vi "Move map.vi"(6 "MAP3":refnum<vi>, 7 "revise":u32=20, 8 "error in":errorcluster, 9 "MAP2":refnum<vi>, 10 "MAP1":refnum<vi>, 11 "Boolean in":refnum<vi>) -> (0 "error out":errorcluster)   [LabVIEW 2010]
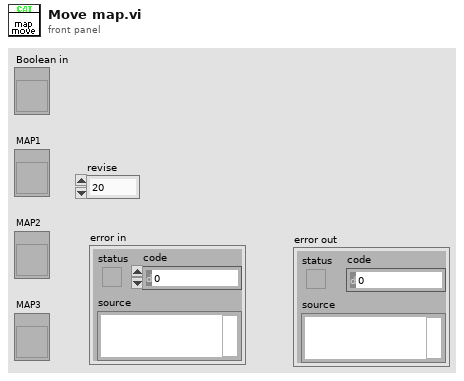
[diagram p1: front panel]
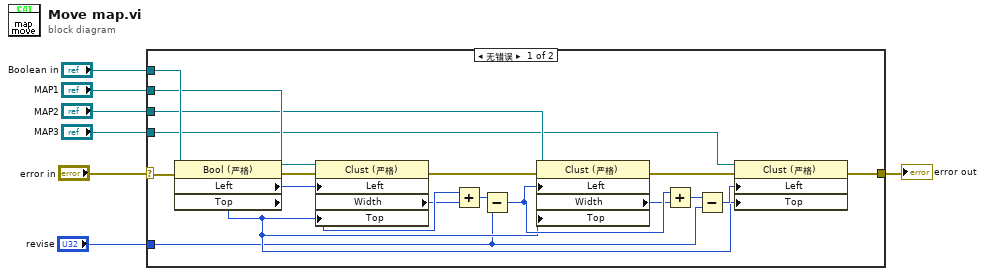
[diagram p0: block diagram]
diagram:
  n1 = case shown="无错误" "error in" {
    selector: "error in" -> [w9 w26]
    tunnel: [w21 w26] -> w7
    tunnel: "Boolean in" -> [w20 _]
    tunnel: "MAP1" -> [w12 _]
    tunnel: "MAP2" -> [w11 _]
    tunnel: "MAP3" -> [w10 _]
    tunnel: "revise" -> [w8 _]
    frame No Error {
      n2 = property class="Bool (严格)"(reference=w20, error in=w9) -> (error out=w15:errorcluster, "Left"=w19:i32, "Top"=w16:i32)  [unwired: 1 out]
      n3 = property class="Clust (严格)"(reference=w12, error in=w15, "Left"=w19, "Top"=w16) -> (error out=w14:errorcluster, "Width"=w18:u32)  [unwired: 1 out]
      n4 = Add(x=w19, y=w18) -> (x+y=w22:u32)
      n5 = Subtract(x=w22, y=w8) -> (x-y=w23:u32)
      n6 = property class="Clust (严格)"(reference=w11, error in=w14, "Left"=w23, "Top"=w16) -> (error out=w13:errorcluster, "Width"=w17:u32)  [unwired: 1 out]
      n7 = Add(x=w23, y=w17) -> (x+y=w24:u32)
      n8 = Subtract(x=w24, y=w8) -> (x-y=w25:u32)
      n9 = property class="Clust (严格)"(reference=w10, error in=w13, "Left"=w25, "Top"=w16) -> (error out=w21:errorcluster)  [unwired: 1 out]
    }
    frame Error {
    }
  }
  "error out" <- w7
